vi "PH_HamamatsuCamera.set Visibility of Cam Attribute Value Set Knobs.vi"(0 "VI in":refnum<vi>, 2 "Parameter":T1=4215968 items=["SENSOR MODE"=4212128, "CCD MODE"=4212384, "READOUT MODE"=4211872, "ACTIVE VIEW INDEX"=4343136, "BITS PER CHANNEL"=4342976, "IMAGE PIXEL TYPE"=4343296, "BINNING"=4215968, "EXPOSURE TIME"=2049184, "CONTRAST GAIN"=3163312, "CONTRAST OFFSET"=3163328, "LIGHT MODE"=2114720, "SENSITIVITY"=2114992, "PHOTON IMAGING MODE"=2115200, "HIGH DYNAMIC RANGE MODE"=3163360, "WHITE BALANCE"=3163568, "TEMPERATURE"=2115232, "TEMPERATURE TARGET"=2115264, "SENSOR COOLER FAN"=2115296, "LINEBUNDLE HEIGHT"=4212192, "MECHANICAL SHUTTER"=2115488, "BACK FOCUS POSITION"=8422304, "TRIGGER CONNECTOR"=1066432, "TRIGGER SOURCE"=1066144, "OUTPUT TRIGGER SOURCE"=1852576, "TRIGGER GLOBAL EXPOSURE"=2049680, "FIRST TRIGGER BEHAVIOR"=2049696, "CHANNEL SYNC"=1852352, "READOUT DIRECTION"=4211904, "PRE HSYNC COUNT"=1852704, "INTERNAL LINE SPEED"=4191408, "INTERNAL LINE INTERVAL"=4191424], 5 "error in (no error)":errorcluster) -> (14 "VI out":refnum<vi>, 19 "error out":errorcluster)   [LabVIEW 2014, in "PH_HamamatsuCamera.lvlib"]
uses:
  PH_HamamatsuCamera.lvlib
  PH_HamamatsuCamera.Cam Parameter.ctl
  PH_Common/PH_Common.lvlib
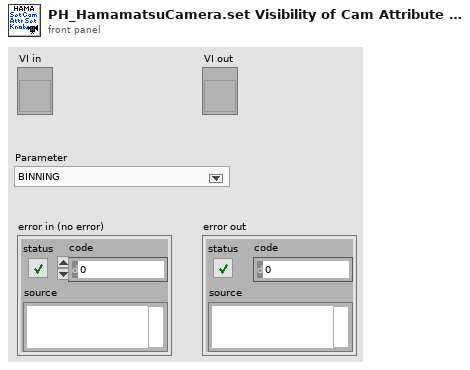
[diagram p1: front panel]
types:
  T1 = typedef "PH_HamamatsuCamera.lvlib/PH_HamamatsuCamera.Cam Parameter.ctl" = u32
  T2 = typedef "PH_HamamatsuCamera.lvlib/PH_HamamatsuCamera.i attribute.ctl" = cluster{"Gui Refs":cluster{"Camera Details":refnum<vi>, "ROI":refnum<vi>, "Set ROI to Maximum":refnum<vi>, "Trigger Parameters":refnum<vi>, "Brightness":refnum<vi>, "Shutter":refnum<vi>, "Gain":refnum<vi>, "Trigger Timeout":refnum<vi>, "Trigger Polarity":refnum<vi>, "Trigger Mode":refnum<vi>, "Parameters":refnum<vi>, "Set Cam Parameter":refnum<vi>, "Parameter to set":refnum<vi>, "Value to set":refnum<vi>}, "Cam":cluster{"Handle":i32, "Details":cluster{"Model":string, "Camera ID":string, "Firmware":string}, "Buffer Info":cluster{"height":u32, "width":u32, "datatype":u32}}, "H Offset":cluster{"Value":i32, "Minimum":i32, "Maximum":i32, "Increment":i32}, "V Offset":cluster{"Value":i32, "Minimum":i32, "Maximum":i32, "Increment":i32}, "H Width":cluster{"Value":i32, "Minimum":i32, "Maximum":i32, "Increment":i32}, "V Width":cluster{"Value":i32, "Minimum":i32, "Maximum":i32, "Increment":i32}, "Trigger Parameters":T3, "Trigger Timeout":u32, "Parameters":T4[], "Indicees Cam Parameters":cluster{"Brightness":i32, "Shutter":i32, "Gain":i32}, "Wanted Values":cluster{"Trigger Settings":T3[], "ROI":T5[], "Parameter":cluster{"Name":string, "Value":dbl}[]}}
  T3 = typedef "PH_HamamatsuCamera.lvlib/PH_HamamatsuCamera.Trigger Parameter.ctl" = cluster{"Mode":u32, "Polarity":u32, "Times":u32, "Delay":dbl}
  T4 = typedef "PH_HamamatsuCamera.lvlib/PH_HamamatsuCamera.Parameter Set.ctl" = cluster{"Parameter":string, "Value":dbl, "Writable":bool, "Range":cluster{"min":dbl, "max":dbl, "step":dbl}, "Default":dbl, "Value Names":cluster{"Name":string, "Value":dbl}[], "Text Values":bool}
  T5 = typedef "PH_HamamatsuCamera.lvlib/PH_HamamatsuCamera.ROI.ctl" = cluster{"Horizontal Offset":i32, "Vertical Offset":i32, "Horizontal Width":i32, "Vertical Width":i32}
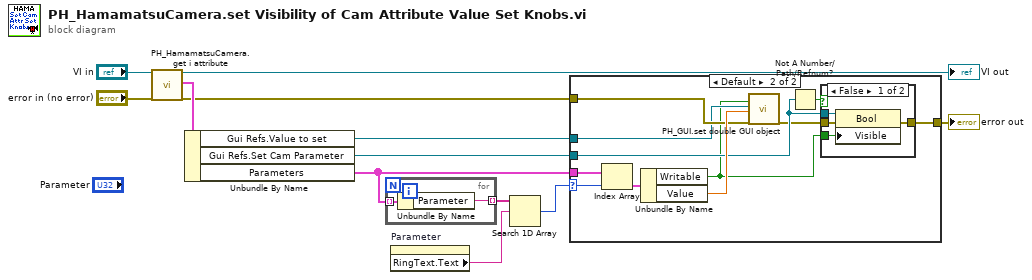
[diagram p0: block diagram]
diagram:
  n1 = call "PH_HamamatsuCamera.get i attribute.vi"("i ref in"="VI in", "error in (no error)"="error in (no error)") -> ("i ref out"=→"VI out":refnum<vi>, "i attribute"=w12:T2, "error out"=w6:errorcluster)  [unwired: 15 in]
  n2 = Unbundle By Name(w12) -> ("Gui Refs.Value to set"=w5:refnum<vi>, "Gui Refs.Set Cam Parameter"=w7:refnum<vi>, "Parameters"=w4:T4[])
  n3 = for {
    tunnel: w4 -> [w14] mode=indexing
    tunnel: [w13] -> w3 mode=indexing
    n4 = Unbundle By Name(w14) -> ("Parameter"=w13:string)
  }
  n5 = property on="Parameter" class="Ring (strict)"() -> ("RingText.Text"=w2:string)  [unwired: 2 in, 2 out]
  n6 = Search 1D Array(1D array=w3, element=w2) -> (index of element=w1:i32)  [unwired: 1 in]
  n7 = case shown="Default" w1 {
    selector: w1 -> [_ w16]
    tunnel: [w15 w24] -> w8
    tunnel: w7 -> [_ w22]
    tunnel: w6 -> [w15 w21]
    tunnel: w5 -> [_ w19]
    tunnel: w4 -> [_ w17]
    frame -1 {
    }
    frame Default {
      n8 = Index Array(array=w17, index=w16) -> (element=w26:T4)
      n9 = Unbundle By Name(w26) -> ("Writable"=w18:bool, "Value"=w23:dbl)
      n10 = call "PH_GUI.set double GUI object.vi"("visible (true)"=w18, "GUI object Ref"=w19, "value"=w23, "error in (no error)"=w21) -> ("error out"=w20:errorcluster)  [unwired: 15 in]
      n11 = Not A Number/Path/Refnum?(number/path/refnum=w22) -> (NaN/Path/Refnum?=w25:bool)
      n12 = case shown="False" w25 {
        tunnel: w18 -> [w30 _]
        tunnel: w20 -> [w29 w31]
        tunnel: [w28 w31] -> w24
        tunnel: w22 -> [w27 _]
        frame False {
          n13 = property on="Property Node" class="Bool"(reference=w27, error in=w29, "Visible"=w30) -> (error out=w28:errorcluster)  [unwired: 1 out]
        }
        frame True {
        }
      }
    }
  }
  "error out" <- w8
